vi "Get Request Type.vi"(8 "error in (no error)":errorcluster, 11 "GetSceneList in":refnum<class "GetSceneList.lvclass">) -> (0 "error out":errorcluster, 2 "Request Type":string, 3 "GetSceneList out":refnum<class "GetSceneList.lvclass">)   [LabVIEW 2022 SP3, in "obs-websocket-lv.lvlib" / "GetSceneList.lvclass"]
uses:
  GetSceneList.lvclass
  GetSceneList.lvclass/GetSceneList.ctl
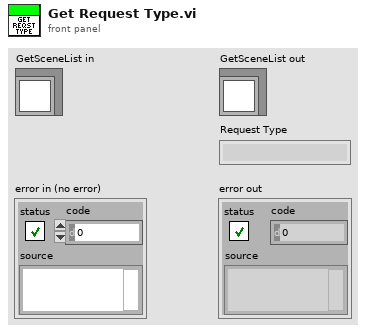
[diagram p1: front panel]
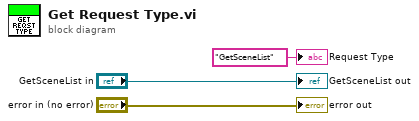
[diagram p0: block diagram]
diagram:
  "error out" <- "error in (no error)"
  "GetSceneList out" <- "GetSceneList in"
  "Request Type" <- "GetSceneList" ("Request Type")
